vi "lab1_event_structure.vi"() -> ()   [LabVIEW 2014]
panel:
  in  "Array":i32[](array[numeric])=[1, 1, 1, 2, 2, 2]
  out "element":i32[](array[numeric])
  in  "Boolean":bool
  in  "stop":bool
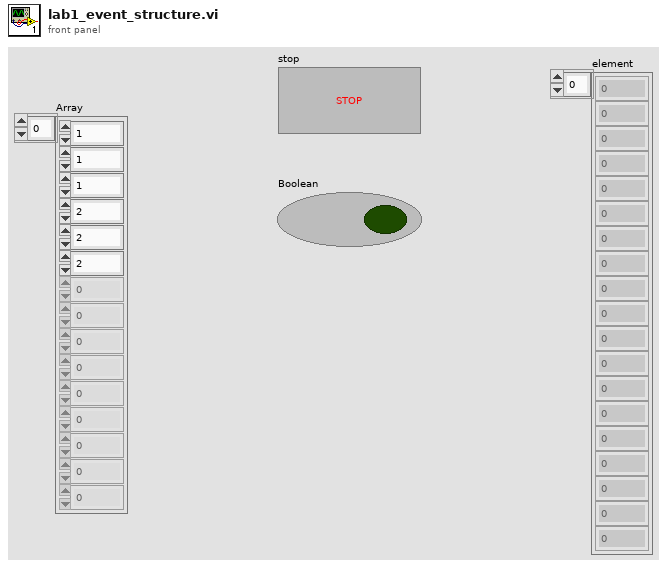
[diagram p1: front panel]
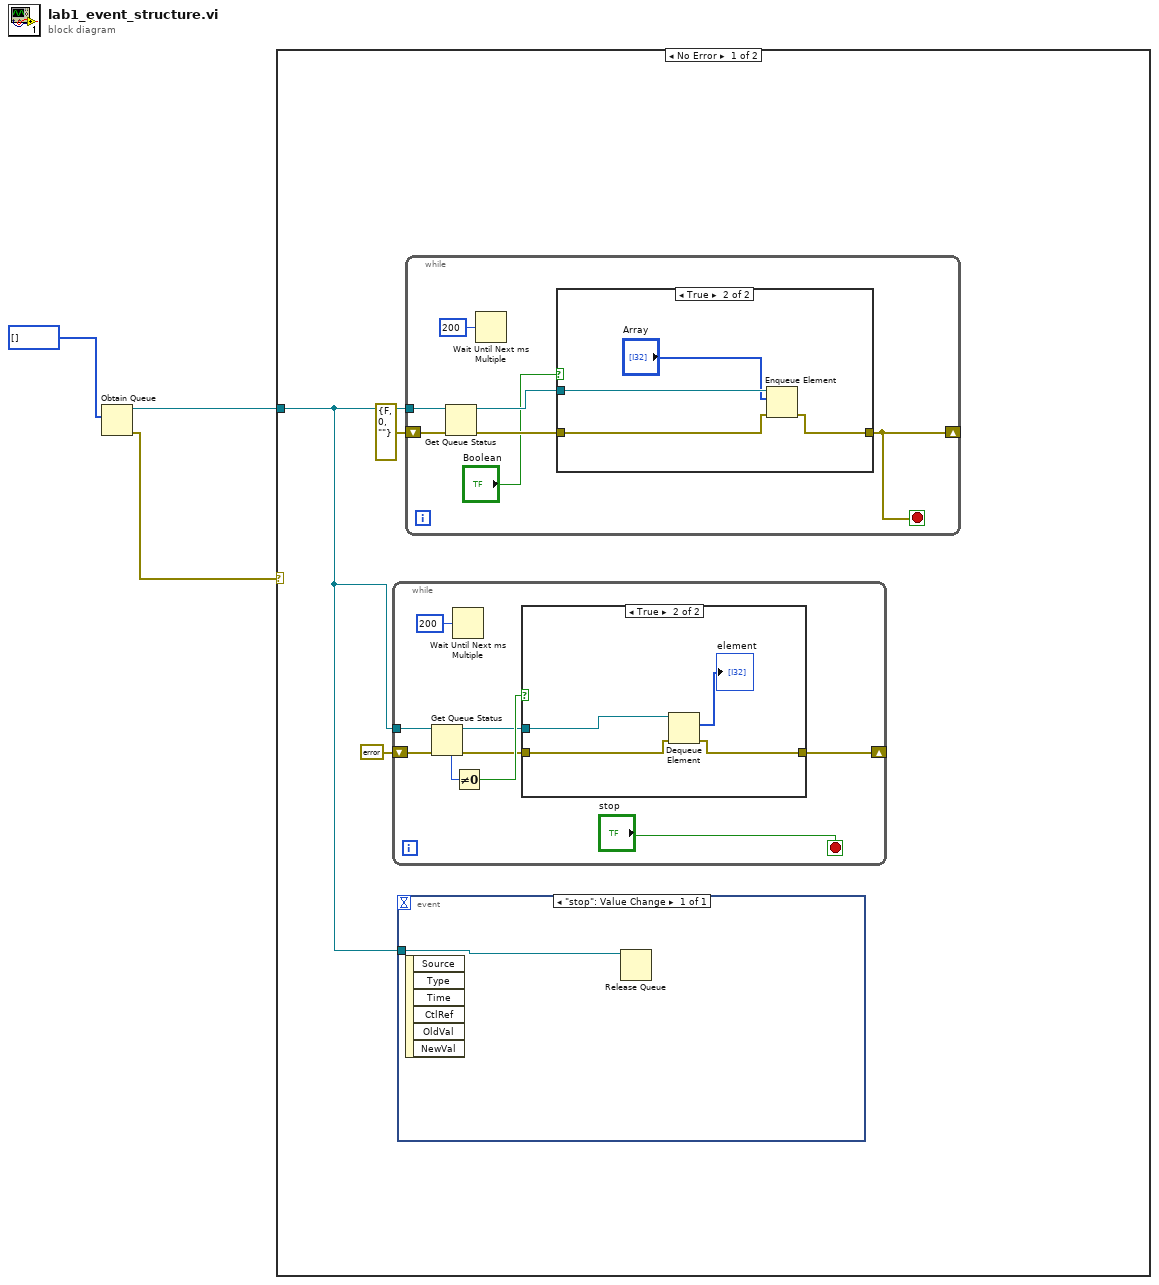
[diagram p0: block diagram]
diagram:
  n1 = Obtain Queue(element data type=i32[] []) -> (queue out=w2:refnum<queue>, error out=w1:errorcluster)  [unwired: 4 in, 1 out]
  n2 = case shown="No Error" w1 {
    tunnel: w2 -> [w4 _]
    frame No Error {
      n3 = while {
        tunnel: w4 -> [w15]
        shift-right: [w9] -> _
        shift-left: errorcluster {"status"=FALSE, "code"=0, "source"=""} ("error out") -> [w10]
        stop <- "stop" stop-if-true
        n4 = Get Queue Status(queue=w15, error in (no error)=w10) -> (queue out=w12:refnum<queue>, error out=w11:errorcluster, # elements in queue=w14:i32)  [unwired: 1 in, 5 out]
        n5 = Wait Until Next ms Multiple(millisecond multiple=u32 200) -> ()  [unwired: 1 out]
        n6 = Not Equal To 0?(x=w14) -> (x != 0?=w13:bool)
        n7 = case shown="True" w13 {
          tunnel: w12 -> [_ w21]
          tunnel: w11 -> [w17 w20]
          tunnel: [w17 w19] -> w9
          frame False {
          }
          frame True {
            n8 = Dequeue Element(queue=w21, error in (no error)=w20) -> (element=→"element":i32[], error out=w19:errorcluster)  [unwired: 1 in, 2 out]
          }
        }
      }
      n9 = event shown="[0] \"stop\": Value Change" {
        selector: _ -> [_]
        dyn-events: _ -> [_]
        timeout: _ -> [_]
        tunnel: w4 -> [w7]
        event "stop": Value Change {
          n10 = event-data() -> ()  [unwired: 1 in, 6 out]
          n11 = Release Queue(queue=w7) -> ()  [unwired: 2 in, 3 out]
        }
      }
      n12 = while {
        tunnel: w4 -> [w28]
        shift-right: [w22] -> _
        shift-left: errorcluster {"status"=FALSE, "code"=0, "source"=""} ("error out") -> [w27]
        stop <- w22 stop-if-true
        n13 = Get Queue Status(queue=w28, error in (no error)=w27) -> (queue out=w25:refnum<queue>, error out=w24:errorcluster)  [unwired: 1 in, 6 out]
        n14 = Wait Until Next ms Multiple(millisecond multiple=u32 200) -> ()  [unwired: 1 out]
        n15 = case shown="True" "Boolean" {
          tunnel: w25 -> [_ w33]
          tunnel: [w29 w32] -> w22
          tunnel: w24 -> [w29 w31]
          frame False {
          }
          frame True {
            n16 = Enqueue Element(queue=w33, element="Array", error in (no error)=w31) -> (error out=w32:errorcluster)  [unwired: 1 in, 2 out]
          }
        }
      }
    }
    frame Error {
    }
  }
